vi "Is External Source.vi"(11 "User BluelinesRedlines in":refnum<class "User BluelinesRedlines.lvclass">) -> (2 "External Source":bool)   [LabVIEW 2020, in "VolatusGUIElements.lvlib" / "User BluelinesRedlines.lvclass"]
uses:
  User BluelinesRedlines.lvclass
  User BluelinesRedlines.lvclass/User BluelinesRedlines.ctl
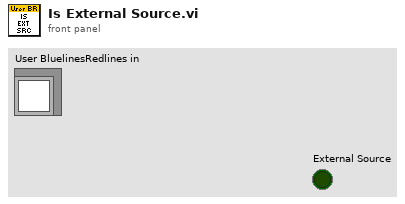
[diagram p1: front panel]
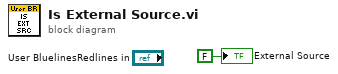
[diagram p0: block diagram]
diagram:
  "External Source" <- FALSE ("External Source")
